vi "Check_EnFlo_Arm.vi"() -> ()   [LabVIEW 2020]
uses:
  Gen Trav/Trav_mode.ctl
  Controls/Home.ctl
  Gen Trav/Route mapping/Route_mapping_global.vi
  Globals/Trav_pos_global.vi
  ADAM Serial/Instrument drivers/Traverses/~subVIs/DriveConfigGlobal.vi
panel:
  out "Position Output XYZ":dbl[](array[numeric]) format="%.2f"
  in  "Mode":T1(ring)
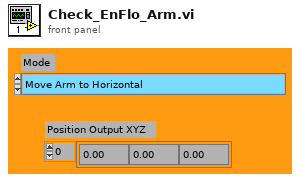
[diagram p1: front panel]
types:
  T1 = enum16{"Move Arm to Horizontal", "Teach Traverse That Arm is Level"}
  T2 = typedef "Tunnel_Coordinates.ctl" = enum16{"Work in Tunnel Coordinates", "Work in Model Coordinates"}
  T3 = typedef "Box_size.ctl" = cluster{"Max":sgl, "Min":sgl}[]
  T4 = typedef "Exclude_cluster.ctl" = cluster{"Sizes":T3, "Name":string, "Exclude Type":T5}
  T5 = typedef "Exclusion_type.ctl" = enum16{"Exclude completely", "Allow only vertical moves"}
  T6 = typedef "Trav_mode.ctl" = enum16{"Move traverse", "Read traverse position", "Teach Position"}
  T7 = enum16{"Load setup from excel file", "Save setup to excel file"}
  T8 = typedef "Home.ctl" = enum16{"Don't Home", "Home  +X", "Home  -X", "Home  +Y", "Home  -Y", "Home  +Z", "Home  -Z"}
  T9 = typedef "AxisConfigCluster.ctl" = cluster{"Channel Properties":T10, "Static Drive Configuration":T11}
  T10 = typedef "DriveProperties.ctl" = cluster{"Channel Name":string, "Vel. Default":sgl, "Acc. Default":sgl, "Vel. Max":sgl, "Vel. Min":sgl, "Acc. Max":sgl, "Acc. Min":sgl, "Pulses/unit":sgl, "Address":u8, "Pulse Offset":i32, "Pos Tolerance":sgl, "Pulses/rev":sgl, "Backlash/Eng units":sgl, "Current Pos":sgl, "Ch Status":enum16{"Active", "Offline", "Simulate"}, "Port Name":string, "Axis Transform mode":string, "Metadata Ch Name":string, "Type":string}
  T11 = typedef "DriveStaticConfig.ctl" = cluster{"Correction Gain % (CG)":u16, "Dead Band (DB)":i32, "Dead Band Window (DW)":i32, "Encoder Resolution (ER)":i32, "Step Mode  (FSB)":u16, "Position Maintenance (FSC)":u16, "Stop on Stall (FSD)":u16, "Activate OP1 on stall (FSE)":u16, "Stop on Trigger 3 (FSF)":u16, "OP2 in Deadband (FSG)":u16, "Stall Detect (FSH)":u16, "Limit Disable (LD)":u16, "Motor Resolution (MR)":enum16{"200", "400", "1000", "2000", "4000", "5000", "10000", "12800", "18000", "20000", "21600", "25000", "25400", "25600", "36000", "50000", "278528", "425984", "507904", "614400", "655360", "819200", "1024000"}, "Limit Switch Sense (OSA)":u16, "Home Position (OSB)":u16, "Home Switch Sense (OSC)":u16, "Encoder Z for Home (OSD)":u16, "Reference edge of Home (OSH)":u16, "RS232 Echo Control (SSA)":u16, "Buffer at Limit (SSG)":u16, "Buffer at Stop (SSH)":u16, "Indexer Mode  (FSA)":u16, "Type":string, "ConfigString":string, "De Power Motor":enum16{"TRUE", "FALSE"}}
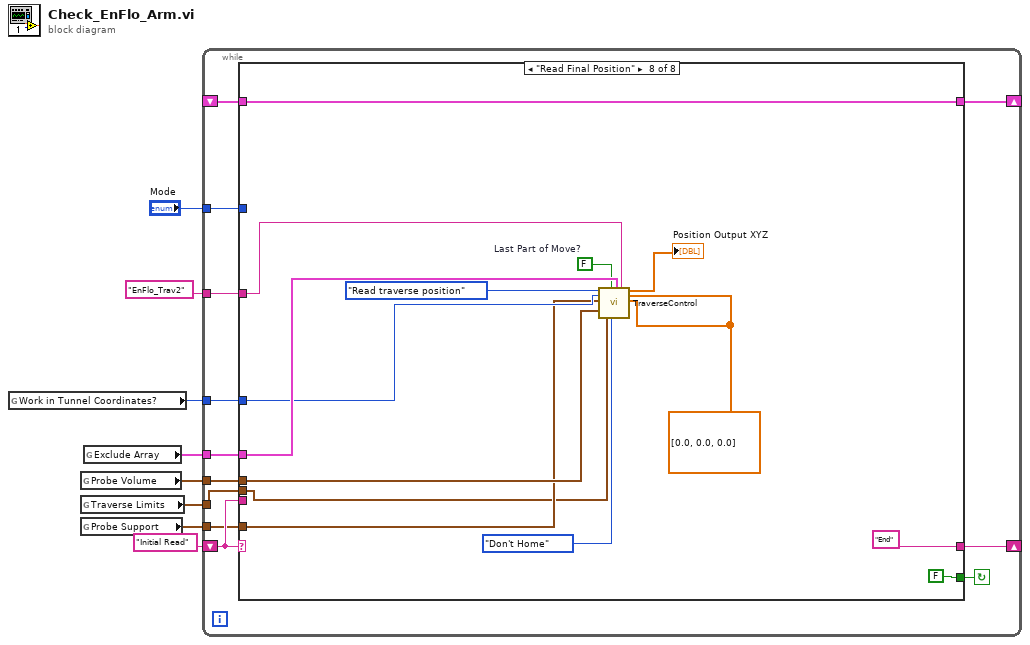
[diagram p0: block diagram]
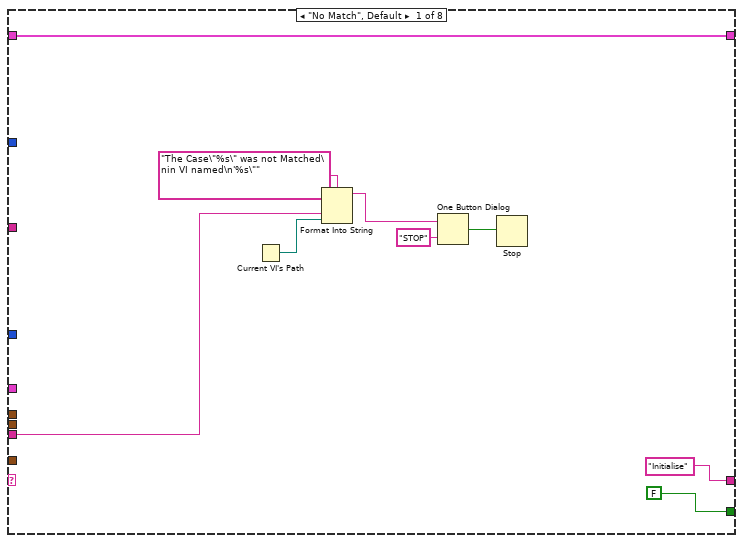
[diagram p2: hidden frame]
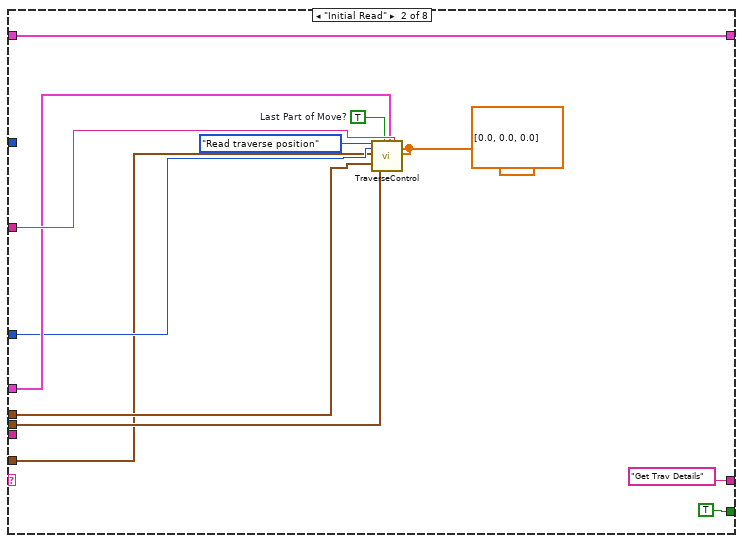
[diagram p3: hidden frame]
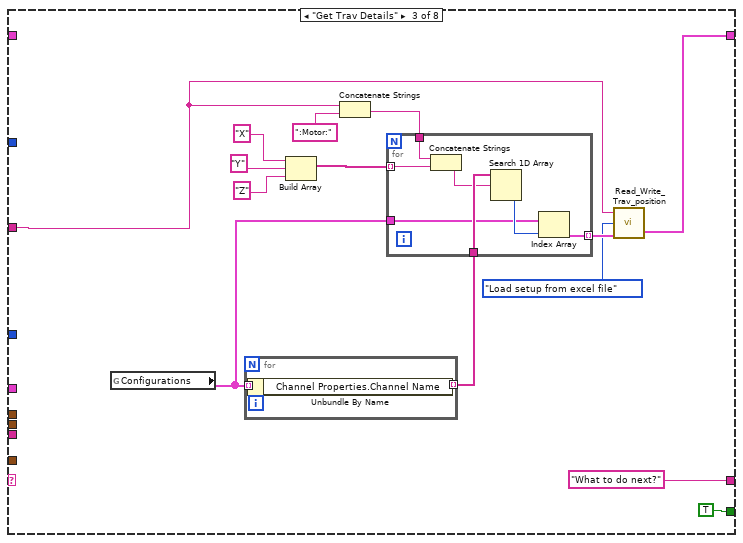
[diagram p4: hidden frame]
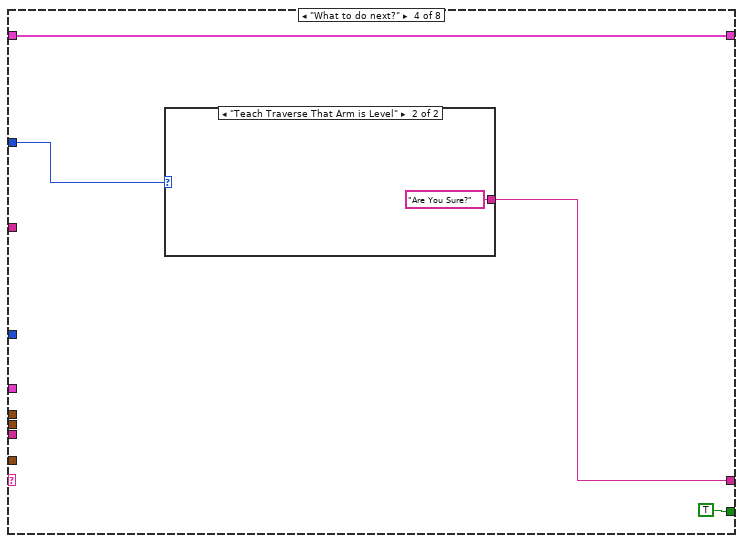
[diagram p5: hidden frame]
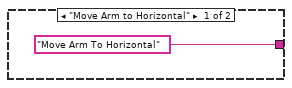
[diagram p6: hidden frame]
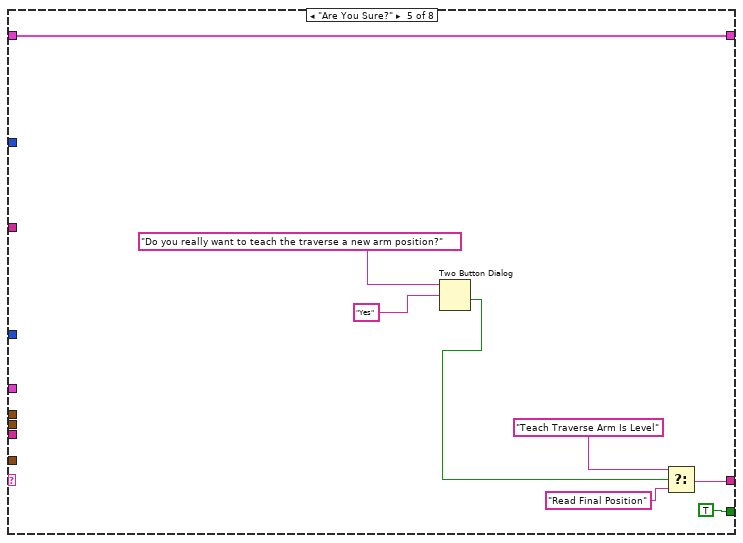
[diagram p7: hidden frame]
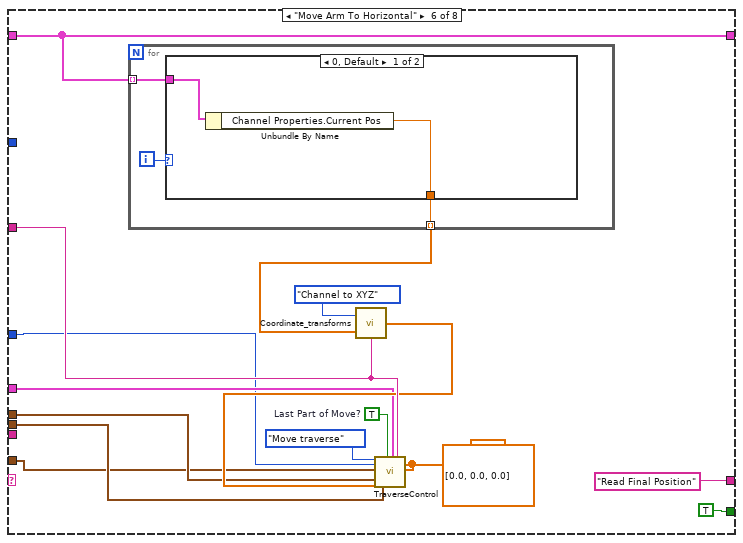
[diagram p8: hidden frame]
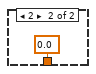
[diagram p9: hidden frame]
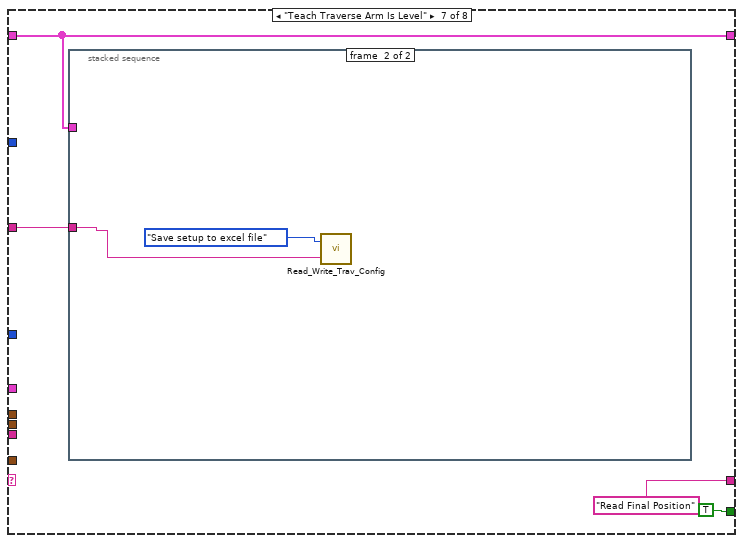
[diagram p10: hidden frame]
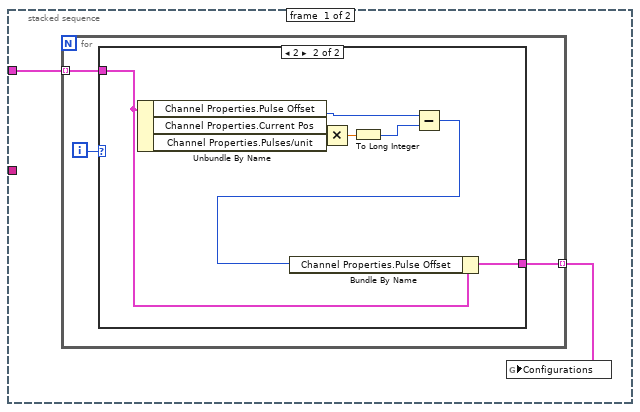
[diagram p11: hidden frame]
diagram:
  n1 = global read "Trav_pos_global.vi" "Work in Tunnel Coordinates?"() -> (w2:T2)
  n2 = global read "Route_mapping_global.vi" "Probe Volume"() -> (w4:T3)
  n3 = global read "Route_mapping_global.vi" "Traverse Limits"() -> (w3:T3)
  n4 = global read "Route_mapping_global.vi" "Probe Support"() -> (w1:T3)
  n5 = global read "Route_mapping_global.vi" "Exclude Array"() -> (w5:T4[])
  n6 = while {
    tunnel: "Mode" -> [w14]
    shift-left: _ -> [w15]
    shift-right: [w16] -> _
    tunnel: "EnFlo_Trav2" ("Traverse Name") -> [w17]
    shift-left: "Initial Read" -> [w18]
    shift-right: [w19] -> _
    tunnel: w5 -> [w13]
    tunnel: w4 -> [w12]
    tunnel: w3 -> [w11]
    tunnel: w2 -> [w10]
    tunnel: w1 -> [w9]
    stop <- w20 continue-if-true
    n7 = case shown="\"Read Final Position\"" w18 {
      tunnel: [FALSE TRUE TRUE TRUE TRUE TRUE TRUE FALSE] -> w20
      tunnel: ["Initialise" "Get Trav Details" "What to do next?" w66 w72 "Read Final Position" "Read Final Position" "End"] -> w19
      tunnel: w18 -> [w24 _ _ _ _ _ _ _]
      tunnel: w17 -> [_ w37 w43 _ _ w88 w100 w130]
      tunnel: [w21 w38 w42 w65 w77 w91 w101 w129] -> w16
      tunnel: w15 -> [w21 w38 _ w65 w77 w91 w101 w129]
      tunnel: w14 -> [_ _ _ w67 _ _ _ _]
      tunnel: w13 -> [_ w36 _ _ _ w85 _ w127]
      tunnel: w12 -> [_ w34 _ _ _ w84 _ w126]
      tunnel: w11 -> [_ w35 _ _ _ w83 _ w121]
      tunnel: w10 -> [_ w33 _ _ _ w82 _ w125]
      tunnel: w9 -> [_ w32 _ _ _ w81 _ w124]
      frame "No Match", Default {
        n8 = Current VI's Path() -> (path=w23:path)
        n9 = Format Into String(format string="The Case\"%s\" was not Matched\nin VI named\n'%s\"" ("Format String"), w24, w23) -> (resulting string=w27:string)  [unwired: 2 in, 1 out]
        n10 = One Button Dialog(message=w27, button name ("OK")="STOP") -> (true=w25:bool)
        n11 = Stop(stop? (T)=w25) -> ()
      }
      frame "Initial Read" {
        w30 = sgl[] [0.0, 0.0, 0.0] ("Trav_Coordinates Current Pos dx;dy;dz")
        w31 = TRUE  # Last Part of Move?
        n12 = call "TraverseControl.vi"("Mode"=Trav_mode."Read traverse position", "Work in Tunnel Coordinates?"=w33, "Probe Support"=w32, "Probe Volume"=w34, "Entire Space"=w35, "Last Part of Move?"=w31, "Exclude Array"=w36, "Traverse Name"=w37, "Trav_Coordinates New Pos dx;dy;dz"=w30, "Trav_Coordinates Current Pos dx;dy;dz"=w30) -> ()  [unwired: 7 in, 3 out]
      }
      frame "Get Trav Details" {
        n13 = global read "DriveConfigGlobal.vi" "Configurations"() -> (w46:T9[])
        n14 = for {
          tunnel: w46 -> [w57] mode=indexing
          tunnel: [w56] -> w47 mode=indexing
          n15 = Unbundle By Name(w57) -> ("Channel Properties.Channel Name"=w56:string)
        }
        n16 = Build Array("X", "Y", "Z") -> (w52:string[])
        n17 = Concatenate Strings(w43, ":Motor:") -> (w51:string)
        n18 = for {
          tunnel: w52 -> [w64] mode=indexing
          tunnel: w51 -> [w63]
          tunnel: w47 -> [w62]
          tunnel: w46 -> [w59]
          tunnel: [w58] -> w45 mode=indexing
          n19 = Concatenate Strings(w63, w64) -> (w61:string)
          n20 = Search 1D Array(1D array=w62, element=w61) -> (index of element=w60:i32)  [unwired: 1 in]
          n21 = Index Array(array=w59, index=w60) -> (element=w58:T9)
        }
        n22 = call "Read_Write_Trav_position.vi"("Matched Configurations In"=w45, "Mode"=T7."Load setup from excel file", "Traverse Name"=w43) -> ("Matched Configurations Out"=w42:T9[])  [unwired: 1 in]
      }
      frame "What to do next?" {
        n23 = case shown="\"Teach Traverse That Arm is Level\"" w67 {
          tunnel: ["Move Arm To Horizontal" "Are You Sure?"] -> w66
          frame "Move Arm to Horizontal" {
          }
          frame "Teach Traverse That Arm is Level" {
          }
        }
      }
      frame "Are You Sure?" {
        n24 = Two Button Dialog(message="Do you really want to teach the traverse a new arm position?", 2:"Yes" ("T button name (\"OK\")")) -> (T button?=w74:bool)  [unwired: 1 in]
        n25 = Select(t="Teach Traverse Arm Is Level", s=w74, f="Read Final Position") -> (s? t:f=w72:string)
      }
      frame "Move Arm To Horizontal" {
        w79 = sgl[] [0.0, 0.0, 0.0] ("Trav_Coordinates Current Pos dx;dy;dz")
        w80 = TRUE  # Last Part of Move?
        n26 = for {
          tunnel: w91 -> [w95] mode=indexing
          tunnel: [w94] -> w89 mode=indexing
          i -> [w96]
          n27 = case shown="0, Default" w96 {
            tunnel: w95 -> [w98 _]
            tunnel: [w97 0.0 ("Current Pos")] -> w94
            frame 0, Default {
              n28 = Unbundle By Name(w98) -> ("Channel Properties.Current Pos"=w97:sgl)
            }
            frame 2 {
            }
          }
        }
        n29 = call "Coordinate_transforms.vi"("Traverse Name"=w88, "Input"=w89, "Mode"=enum16{"XYZ to Channel", "Channel to XYZ"}."Channel to XYZ") -> ("Output"=w87:sgl[])
        n30 = call "TraverseControl.vi"("Mode"=Trav_mode."Move traverse", "Work in Tunnel Coordinates?"=w82, "Probe Support"=w81, "Probe Volume"=w84, "Position input XYZ"=w87, "Entire Space"=w83, "Last Part of Move?"=w80, "Exclude Array"=w85, "Traverse Name"=w88, "Trav_Coordinates New Pos dx;dy;dz"=w79, "Trav_Coordinates Current Pos dx;dy;dz"=w79) -> ()  [unwired: 6 in, 3 out]
      }
      frame "Teach Traverse Arm Is Level" {
        n31 = stacked-sequence {
          tunnel: w101 -> [w105 _]
          tunnel: w100 -> [_ w118]
          frame #0 {
            n32 = for {
              tunnel: w105 -> [w107] mode=indexing
              tunnel: [w106] -> w104 mode=indexing
              i -> [w108]
              n33 = case shown="2" w108 {
                tunnel: w107 -> [w109 w114]
                tunnel: [w109 w110] -> w106
                frame 0, Default {
                }
                frame 2 {
                  n34 = Unbundle By Name(w114) -> ("Channel Properties.Pulse Offset"=w115:i32, "Channel Properties.Current Pos"=w117:sgl, "Channel Properties.Pulses/unit"=w116:sgl)
                  n35 = Multiply(x=w117, y=w116) -> (x*y=w113:sgl)
                  n36 = To Long Integer(number=w113) -> (32bit integer=w112:i32)
                  n37 = Subtract(x=w115, y=w112) -> (x-y=w111:i32)
                  n38 = Bundle By Name(cluster=w114, "Channel Properties.Pulse Offset"=w111) -> (w110:T9)
                }
              }
            }
            n39 = global write "DriveConfigGlobal.vi" "Configurations"(w104) -> ()
          }
          frame #1 {
            n40 = call "Read_Write_Trav_Config.vi"("Traverse Name"=w118, "Mode"=T7."Save setup to excel file") -> ()  [unwired: 1 out]
          }
        }
      }
      frame "Read Final Position" {
        w120 = sgl[] [0.0, 0.0, 0.0] ("Trav_Coordinates Current Pos dx;dy;dz")
        w122 = FALSE  # Last Part of Move?
        n41 = call "TraverseControl.vi"("Mode"=Trav_mode."Read traverse position", "Work in Tunnel Coordinates?"=w125, "Probe Support"=w124, "Probe Volume"=w126, "Entire Space"=w121, "Last Part of Move?"=w122, "Home"=Home."Don't Home", "Exclude Array"=w127, "Traverse Name"=w130, "Trav_Coordinates New Pos dx;dy;dz"=w120, "Trav_Coordinates Current Pos dx;dy;dz"=w120) -> ("Position Output XYZ"=→"Position Output XYZ":sgl[])  [unwired: 6 in, 2 out]
      }
    }
  }
